vi "updateCol4ColorWhenLoading.vi"(8 "error in":errorcluster, 9 "rowNum":i32, 10 "judgeRes":string, 11 "Tbl Refnum in":refnum<vi>) -> (0 "error out":errorcluster, 3 "Tbl Refnum Out":refnum<vi>)   [LabVIEW 2010]
uses:
  <vilib>/Utility/miscctls.llb/LVRowAndColumnTypeDef.ctl
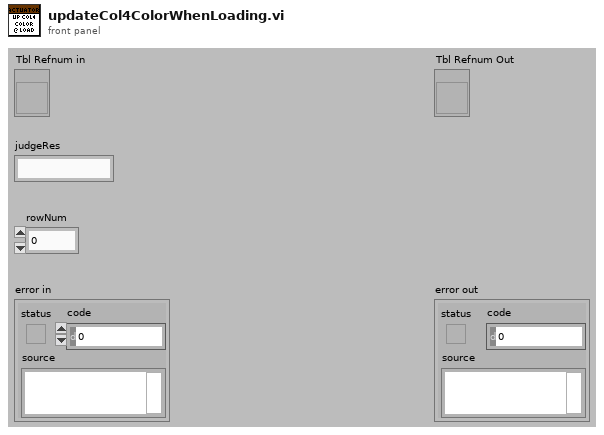
[diagram p1: front panel]
types:
  T1 = typedef "LVRowAndColumnTypeDef.ctl" = cluster{"Row":i32, "Column":i32}
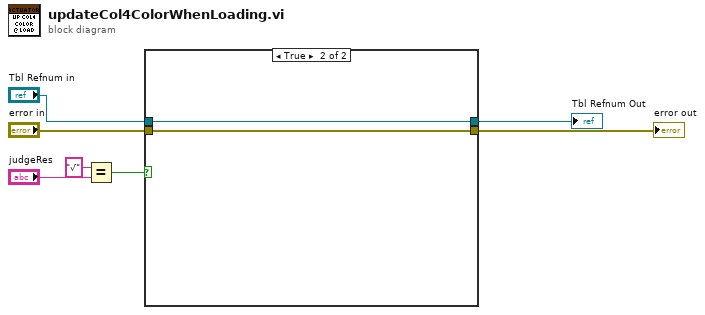
[diagram p0: block diagram]
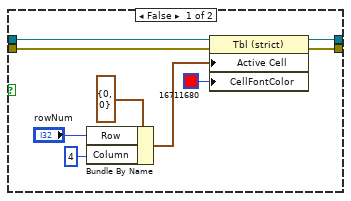
[diagram p2: hidden frame]
diagram:
  n1 = Equal?(x="√", y="judgeRes") -> (x = y?=w5:bool)
  n2 = case shown="True" w5 {
    tunnel: "error in" -> [w11 w17]
    tunnel: "Tbl Refnum in" -> [w10 w18]
    tunnel: [w9 w18] -> w2
    tunnel: [w8 w17] -> w1
    frame False {
      n3 = Bundle By Name(cluster=T1 {"Row"=0, "Column"=0} ("Active Cell:Active Cell"), "Row"="rowNum", "Column"=4) -> (w14:T1)
      n4 = property on="Property Node" class="Tbl (strict)"(reference=w10, error in=w11, "Active Cell"=w14, "CellFontColor"=u32 16711680) -> (reference out=w9:refnum<vi>, error out=w8:errorcluster)
    }
    frame True {
    }
  }
  "Tbl Refnum Out" <- w2
  "error out" <- w1
